vi "Update Time.vi"(8 "error in (no error)":errorcluster, 10 "Timestamp":timestamp, 11 "Example Sink In":refnum<class "Alternative Example Sink.lvclass">) -> (0 "error out":errorcluster, 3 "Example Sink Out":refnum<class "Alternative Example Sink.lvclass">)   [LabVIEW 2016, in "Alternative Example Sink.lvlib" / "Alternative Example Sink.lvclass"]
uses:
  Alternative Example Sink.lvclass
  Alternative Example Sink.lvclass/Alternative Example Sink.ctl
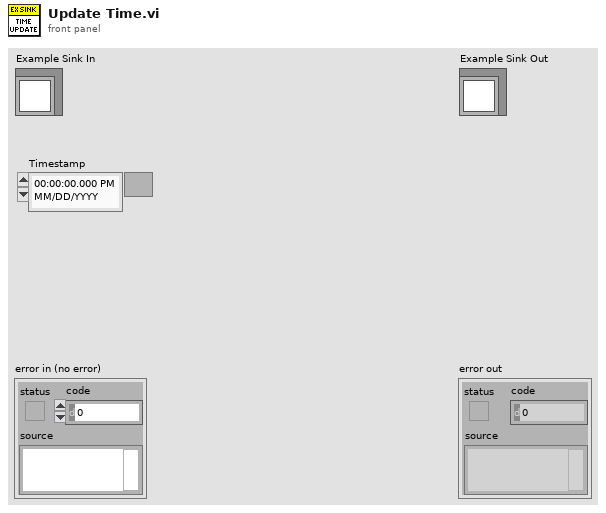
[diagram p1: front panel]
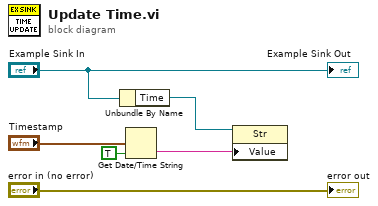
[diagram p0: block diagram]
diagram:
  n1 = Unbundle By Name("Example Sink In") -> ("Time"=w4:refnum<vi>)
  n2 = Get Date/Time String(seconds (now)="Timestamp", want seconds? (F)=TRUE) -> (time string=w3:string)  [unwired: 1 in, 1 out]
  n3 = property class="Str"(reference=w4, "Value"=w3) -> ()  [unwired: 1 in, 2 out]
  "error out" <- "error in (no error)"
  "Example Sink Out" <- "Example Sink In"
